vi "test_F9P_ubx_gmap.vi"() -> ()   [LabVIEW 2019]
uses:
  C:/Users/WEGO/Documents/GitHub/Ycar/LabVIEW/Gmap/dll/GMap.NET.WindowsForms.dll
  Gmap/dll/GMap.NET.WindowsForms.dll
  Ctrl/gnss_config.ctl
  Ctrl/ublox-ui_main.ctl
  Ctrl/ublox_ubx-format.ctl
  Ctrl/ubx-packet.ctl
  Ctrl/cmd_common.ctl
  Gmap/gmap_fgv-cmd.ctl
  Gmap/marker_info.ctl
panel:
  in  "GNSS":enum32{"MainUI", "Data "}(tab)
  in  "gmap center":bool
  in  "zoom":dbl(slide) scale=3.0..20.0
  in  "PinDropMrkr":T1(ring)=enum."red_dot" caption="Pin Drop Marker"
  in  "Lon":dbl format="%.11f"
  in  "Lat Dbclk":dbl format="%.11f"
  in  "Lon Dbclk":dbl format="%.11f"
  in  "Lat":dbl format="%.11f"
  in  "GNSS cfg":T2={"Port"="COM10", "heading select"="", "PwrPak7_mode select"=[], "rate"=115200}
  out "LatLong_nmea":cluster{dbl, dbl} {"?" format="%.9f"; "?" format="%.9f"}
  in  "GMapControl":refnum<k24>(container)
  out "MainUI_gnss":T3 {"HDOP" scale=0.0..10.0; "PDOP" scale=0.0..10.0; "2D Acc.m" scale=0.0..10.0; "Latitude" format="%.8f"; "Longitude" format="%.8f"; "3D Acc.m" scale=0.0..10.0}
  out "rx all":string
  in  "stop":bool
  out "latlong_ubx":cluster{dbl, dbl} {"?" format="%.8f"; "?" format="%.8f"}
  in  "GxGGA latlong":bool
  out "error out":errorcluster
  out "buffer n":u32(graph)
  out "ubx arr":T4 {"payload" format="%02x"; "chksum" format="%02x"; "next" format="%02x"}
  out "rx ubx":string
  out "rx val":string
  # "U-center beta with LabVIEW"
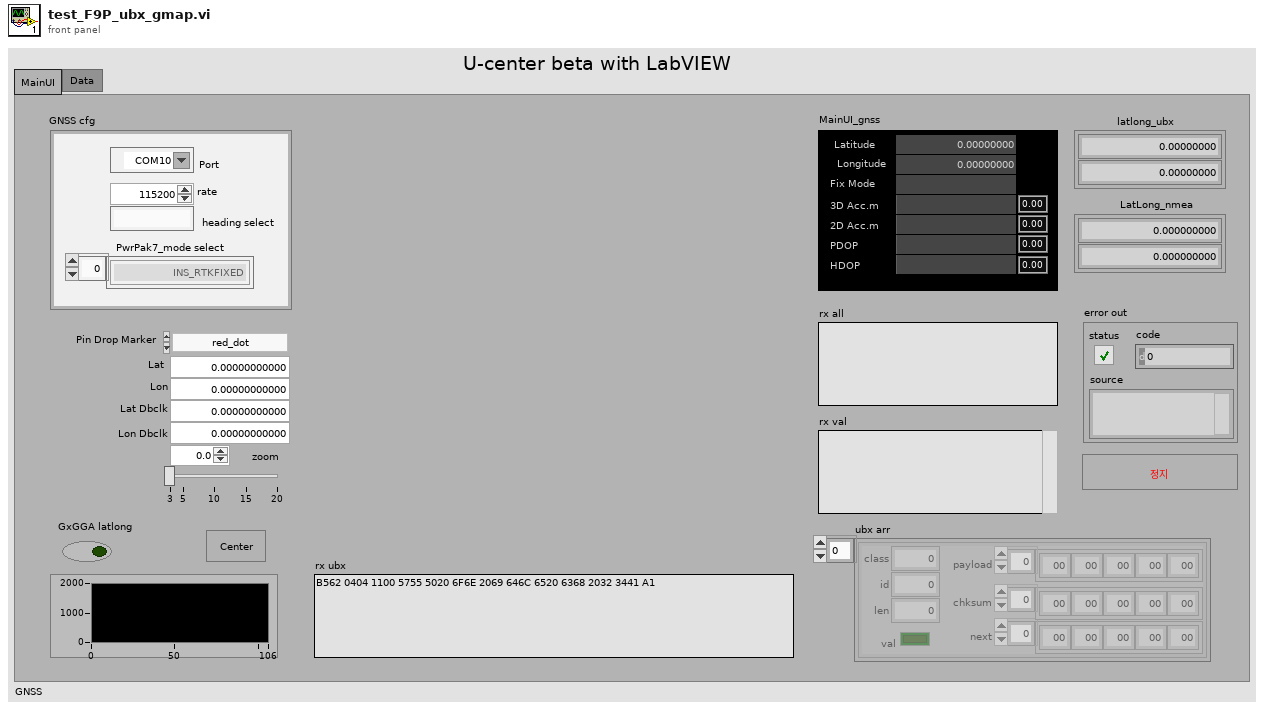
[diagram p1: front panel]
types:
  T1 = enum16{"none", "arrow", "blue", "blue_small", "blue_dot", "blue_pushpin", "brown_small", "gray_small", "green", "green_small", "green_dot", "green_pushpin", "green_big_go", "yellow", "yellow_small", "yellow_dot", "yellow_big_pause", "yellow_pushpin", "lightblue", "lightblue_dot", "lightblue_pushpin", "orange", "orange_small", "orange_dot", "pink", "pink_dot", "pink_pushpin", "purple", "purple_small", "purple_dot", "purple_pushpin", "red", "red_small", "red_dot", "red_pushpin", "red_big_stop", "black_small", "white_small"}
  T2 = typedef "gnss_config.ctl" = cluster{"Port":refnum<visa-resource-name>, "heading select":string, "PwrPak7_mode select":string[], "rate":u32}
  T3 = typedef "ublox-ui_main.ctl" = cluster{"Latitude":dbl, "Longitude":dbl, "Fix Mode":string, "3D Acc.m":dbl, "2D Acc.m":dbl, "PDOP":dbl, "HDOP":dbl}
  T4 = typedef "ublox_ubx-format.ctl" = T5[]
  T5 = typedef "ubx-packet.ctl" = cluster{"class":u8, "id":u8, "len":u8, "payload":u8[], "chksum":u8[], "next ":u8[], "val":bool}
  T6 = typedef "cmd_common.ctl" = enum16{"read", "write"}
  T7 = cluster{"Lat":refnum<vi>, "Lon":refnum<vi>, "Lat Dbclk":refnum<vi>, "Lon Dbclk":refnum<vi>, "zoom":refnum<vi>, "PinDropMrkr":refnum<vi>}
  T8 = typedef "gmap_fgv-cmd.ctl" = enum16{"marker type change", "save_image", "coll of points", "zoom n center markers", "add overlay reference", "read", "zoom", "set position by keyword", "set map provider", "map provider update", "create", "add marker", "clear marker", "close"}
  T9 = enum16{"GxDTM", "GxGBS", "GxGGA", "GxGLL", "GxGNS", "GxGRS", "GxGSA", "GxGST", "GxGSV", "GxRLM", "GxRMC", "GxTHS", "GxTXT", "GxVLW", "GxVTG", "GxZDA"}
  T10 = typedef "marker_info.ctl" = cluster{"arrLatLngActv":dbl[], "type":i32}
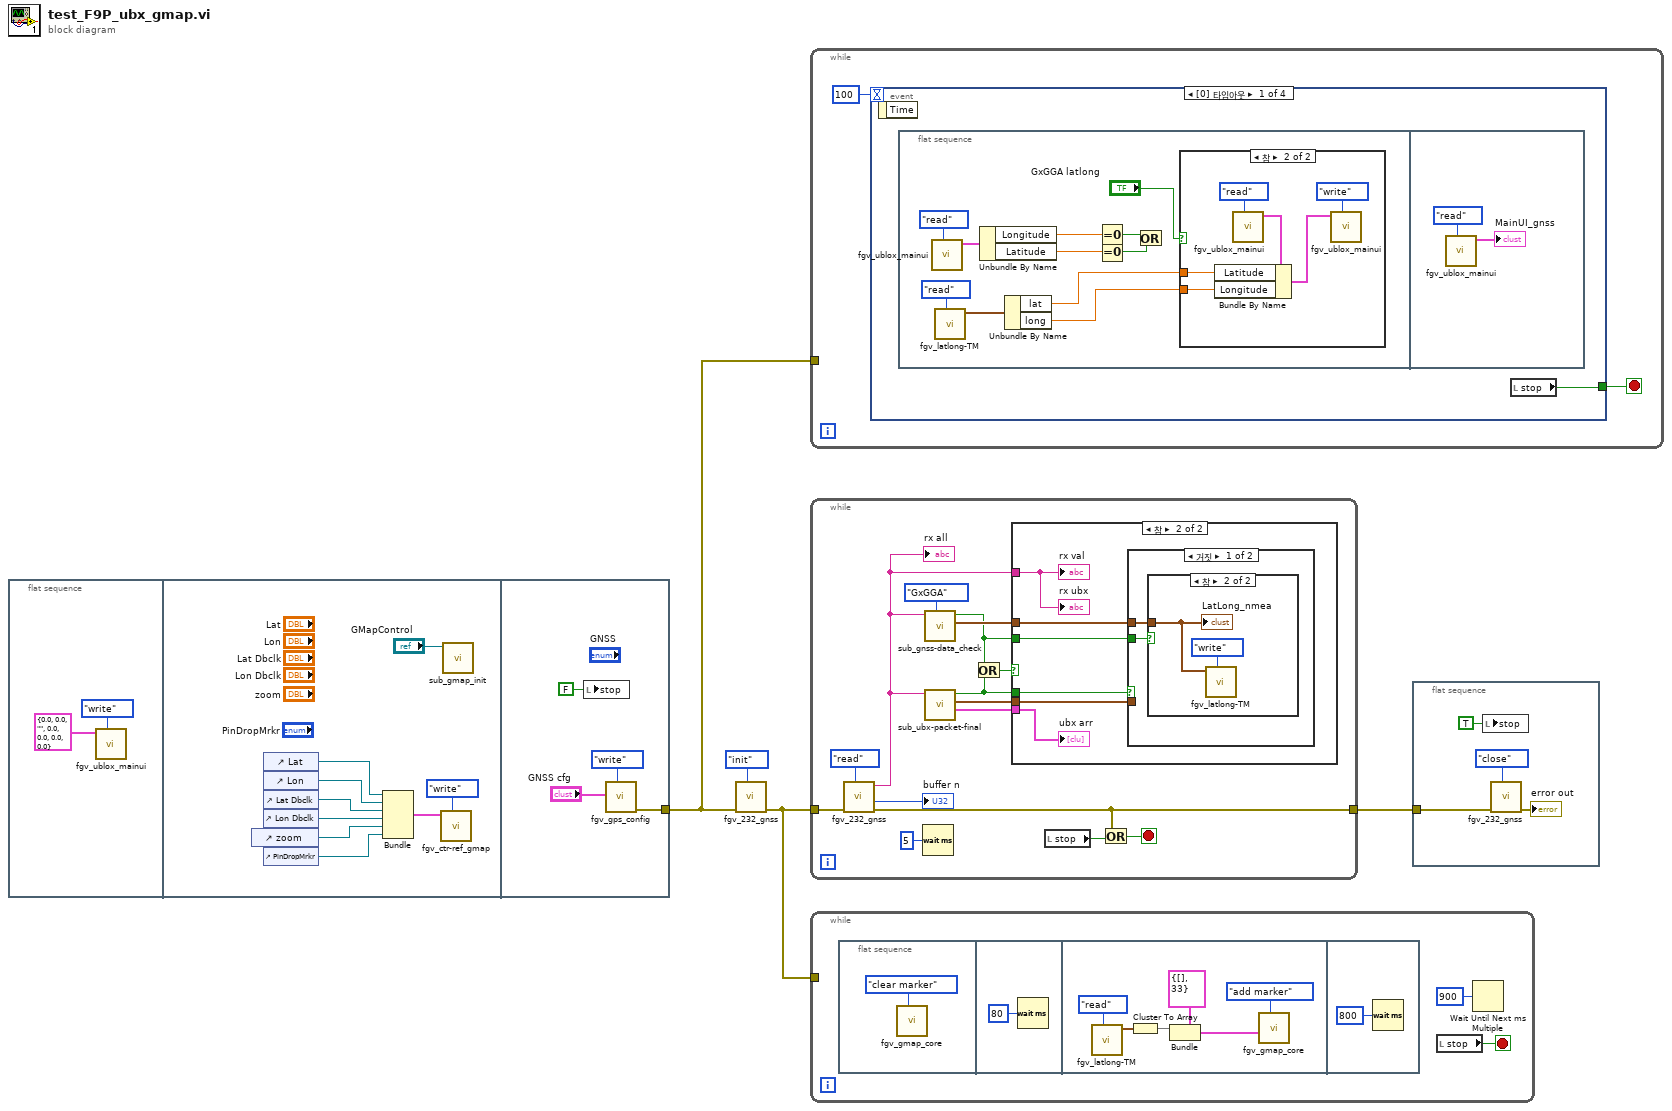
[diagram p0: block diagram]
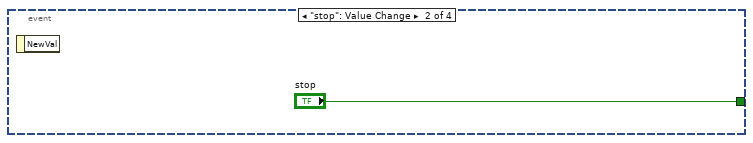
[diagram p3: hidden frame]
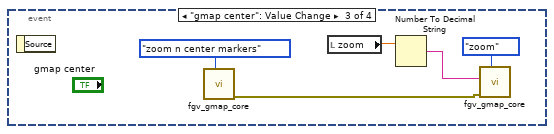
[diagram p4: hidden frame]
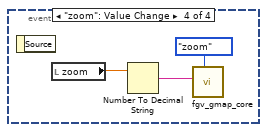
[diagram p5: hidden frame]
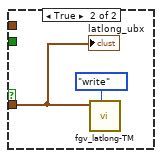
[diagram p8: hidden frame]
diagram:
  n1 = flat-sequence {
    tunnel: [w18] -> w1
    frame #0 {
      n2 = call "fgv_ublox_mainui.vi"("cmd"=cmd_common."write", "MainUI ublox"=T3 {"Latitude"=0.0, "Longitude"=0.0, "Fix Mode"="", "3D Acc.m"=0.0, "2D Acc.m"=0.0, "PDOP"=0.0, "HDOP"=0.0}) -> ()  [unwired: 9 in, 1 out]
    }
    frame #1 {
      n3 = control-ref of="zoom"() -> (w8:refnum<vi>)
      n4 = control-ref of="Lat"() -> (w12:refnum<vi>)
      n5 = control-ref of="Lon"() -> (w11:refnum<vi>)
      n6 = control-ref of="Lat Dbclk"() -> (w10:refnum<vi>)
      n7 = control-ref of="Lon Dbclk"() -> (w9:refnum<vi>)
      n8 = control-ref of="PinDropMrkr"() -> (w7:refnum<vi>)
      n9 = Bundle("Lat"=w12, "Lon"=w11, "Lat Dbclk"=w10, "Lon Dbclk"=w9, "zoom"=w8, "PinDropMrkr"=w7) -> (w14:T7)  [unwired: 1 in]
      n10 = call "fgv_ctr-ref_gmap.vi"("cmd"=cmd_common."write", "ref in"=w14) -> ()  [unwired: 9 in, 1 out]
      n11 = call "sub_gmap_init.vi"("GMapControl"="GMapControl") -> ()  [unwired: 10 in, 1 out]
    }
    frame #2 {
      n12 = local write "stop"(FALSE ("정지")) -> ()
      n13 = call "fgv_gps_config.vi"("cmd"=enum16{"read", "write"}."write", "GNSS cfg"="GNSS cfg") -> ("error out"=w18:errorcluster)  [unwired: 8 in, 1 out]
    }
  }
  n14 = call "fgv_232_gnss.vi"("cmd"=enum16{"init", "read", "write", "close"}."init", "error in"=w1) -> ("error out"=w2:errorcluster)  [unwired: 7 in, 2 out]
  n15 = while {
    tunnel: w1 -> [_]
    stop <- w21 stop-if-true
    n16 = event shown="[0] 타임아웃" {
      selector: _ -> [_ _ _ _]
      dyn-events: _ -> [_ _ _ _]
      timeout: 100 -> [_ _ _ _]
      tunnel: [w22 "stop" _ _] -> w21
      event Timeout {
        n17 = event-data() -> ()  [unwired: 1 in, 1 out]
        n18 = flat-sequence {
          frame #0 {
            n19 = call "fgv_ublox_mainui.vi"("cmd"=cmd_common."read") -> ("MainUI ublox out"=w32:T3)  [unwired: 10 in]
            n20 = call "fgv_latlong-TM.vi"("cmd"=enum16{"write", "read"}."read") -> ("latlong out"=w26:cluster{"lat":dbl, "long":dbl})  [unwired: 9 in, 1 out]
            n21 = Unbundle By Name(w32) -> ("Longitude"=w29:dbl, "Latitude"=w28:dbl)
            n22 = Unbundle By Name(w26) -> ("lat"=w25:dbl, "long"=w24:dbl)
            n23 = Equal To 0?(x=w29) -> (x = 0?=w31:bool)
            n24 = Equal To 0?(x=w28) -> (x = 0?=w30:bool)
            n25 = Or(x=w31, y=w30) -> ()  [unwired: 1 out]
            n26 = case shown="참" "GxGGA latlong" {
              tunnel: w25 -> [_ w35]
              tunnel: w24 -> [_ w34]
              frame False {
              }
              frame True {
                n27 = call "fgv_ublox_mainui.vi"("cmd"=cmd_common."read") -> ("MainUI ublox out"=w38:T3)  [unwired: 10 in]
                n28 = Bundle By Name(cluster=w38, "Latitude"=w35, "Longitude"=w34) -> (w39:T3)
                n29 = call "fgv_ublox_mainui.vi"("cmd"=cmd_common."write", "MainUI ublox"=w39) -> ()  [unwired: 9 in, 1 out]
              }
            }
          }
          frame #1 {
            n30 = call "fgv_ublox_mainui.vi"("cmd"=cmd_common."read") -> ("MainUI ublox out"=→"MainUI_gnss":T3)  [unwired: 10 in]
          }
        }
        n31 = local read "stop"() -> (w22:bool)
      }
      event "stop": Value Change {
        n32 = event-data() -> ()  [unwired: 1 in, 1 out]
      }
      event "gmap center": Value Change {
        n33 = event-data() -> ()  [unwired: 1 in, 1 out]
        n34 = call "fgv_gmap_core.vi"("cmd"=gmap_fgv-cmd."zoom n center markers") -> ("error out"=w43:errorcluster)  [unwired: 7 in, 3 out]
        n35 = local read "zoom"() -> (w46:dbl)
        n36 = Number To Decimal String(number=w46) -> (decimal integer string=w45:string)  [unwired: 1 in]
        n37 = call "fgv_gmap_core.vi"(7:"cmd"=gmap_fgv-cmd."zoom" ("cmd"), "error in"=w43, 10:"cmd"=w45) -> ()  [unwired: 5 in, 4 out]
      }
      event "zoom": Value Change {
        n38 = event-data() -> ()  [unwired: 1 in, 1 out]
        n39 = local read "zoom"() -> (w49:dbl)
        n40 = Number To Decimal String(number=w49) -> (decimal integer string=w48:string)  [unwired: 1 in]
        n41 = call "fgv_gmap_core.vi"(7:"cmd"=gmap_fgv-cmd."zoom" ("cmd"), 10:"cmd"=w48) -> ()  [unwired: 6 in, 4 out]
      }
    }
  }
  n42 = while {
    tunnel: w2 -> [w63]
    tunnel: [w60] -> w3
    stop <- w59 stop-if-true
    n43 = call "fgv_232_gnss.vi"("cmd"=enum16{"init", "read", "write", "close"}."read", "error in"=w63) -> ("error out"=w60:errorcluster, "byte n"=→"buffer n":u32, "read_buffer"=w57:string)  [unwired: 7 in]
    "rx all" <- w57
    n44 = Wait (ms)(milliseconds to wait=u32 5 ("대기 시간 (ms)")) -> ()  [unwired: 1 out]
    n45 = call "sub_gnss-data_check.vi"("sel"=T9."GxGGA", "gnss str"=w57) -> ("LatLong"=w52:cluster{dbl, dbl}, "val"=w51:bool)  [unwired: 7 in, 1 out]
    n46 = call "sub_ubx-packet-final.vi"("read_buffer"=w57) -> ("ubx arr"=w54:T5[], "latlong"=w55:cluster{dbl, dbl}, "val"=w53:bool)  [unwired: 8 in]
    n47 = Or(x=w51, y=w53) -> (x .or. y?=w56:bool)
    n48 = case shown="참" w56 {
      tunnel: w52 -> [_ w66]
      tunnel: w57 -> [_ w70]
      tunnel: w55 -> [_ w67]
      tunnel: w54 -> [_ w71]
      tunnel: w53 -> [_ w69]
      tunnel: w51 -> [_ w68]
      frame False {
      }
      frame True {
        n49 = case shown="거짓" w69 {
          tunnel: w68 -> [w73 _]
          tunnel: w67 -> [_ w76]
          tunnel: w66 -> [w72 _]
          frame False {
            n50 = case shown="참" w73 {
              tunnel: w72 -> [_ w74]
              frame False {
              }
              frame True {
                n51 = call "fgv_latlong-TM.vi"("cmd"=enum16{"write", "read"}."write", "latlong"=w74) -> ()  [unwired: 8 in, 2 out]
                "LatLong_nmea" <- w74
              }
            }
          }
          frame True {
            n52 = call "fgv_latlong-TM.vi"("cmd"=enum16{"write", "read"}."write", "latlong"=w76) -> ()  [unwired: 8 in, 2 out]
            "latlong_ubx" <- w76
          }
        }
        "rx val" <- w70
        "rx ubx" <- w70
        "ubx arr" <- w71
      }
    }
    n53 = local read "stop"() -> (w61:bool)
    n54 = Or(x=w60, y=w61) -> (x .or. y?=w59:bool)
  }
  n55 = while {
    tunnel: w2 -> [_]
    stop <- w79 stop-if-true
    n56 = flat-sequence {
      frame #0 {
        n57 = call "fgv_gmap_core.vi"("cmd"=gmap_fgv-cmd."clear marker") -> ()  [unwired: 7 in, 4 out]
      }
      frame #1 {
        n58 = Wait (ms)(milliseconds to wait=u32 80 ("대기 시간 (ms)")) -> ()  [unwired: 1 out]
      }
      frame #2 {
        n59 = call "fgv_latlong-TM.vi"("cmd"=enum16{"write", "read"}."read") -> ("latlong out"=w82:cluster{"lat":dbl, "long":dbl})  [unwired: 9 in, 1 out]
        n60 = Cluster To Array(cluster=w82) -> (array=w86:dbl[])
        n61 = Bundle(cluster=T10 {"arrLatLngActv"=[], "type"=33} ("marker_info"), "arrLatLngActv"=w86) -> (w84:T10)  [unwired: 1 in]
        n62 = call "fgv_gmap_core.vi"("cmd"=gmap_fgv-cmd."add marker", "marker_info"=w84) -> ()  [unwired: 6 in, 4 out]
      }
      frame #3 {
        n63 = Wait (ms)(milliseconds to wait=u32 800 ("대기 시간 (ms)")) -> ()  [unwired: 1 out]
      }
    }
    n64 = local read "stop"() -> (w79:bool)
    n65 = Wait Until Next ms Multiple(millisecond multiple=u32 900 ("ms 배수")) -> ()  [unwired: 1 out]
  }
  n66 = flat-sequence {
    tunnel: w3 -> [w91]
    frame #0 {
      n67 = local write "stop"(TRUE ("stop")) -> ()
      n68 = call "fgv_232_gnss.vi"("cmd"=enum16{"init", "read", "write", "close"}."close", "error in"=w91) -> ("error out"=→"error out":errorcluster)  [unwired: 7 in, 2 out]
    }
  }
